vi "Read (Waveform).vi"(5 "Bind Source Channel (2: None)":i32(ring)=2 items=["Sub Source 0", "Sub Source 1", "None"], 7 "Probe atenuation":dbl format="%#_13g", 8 "error in (no error)":errorcluster, 9 "Timeout (10000 ms)":u32=10000, 10 "Source (0: Channel 1)":u16(ring) items=["Channel 1", "Channel 2", "Channel 3", "Channel 4", "Math", "Reference A", "Reference B", "Reference C", "Reference D", "FFT"], 11 "KS EDU-X 1002G in":refnum<class "KS EDU-X 1002G.lvclass">) -> (0 "error out":errorcluster, 2 "Waveform Data":waveform(dbl)(graph), 3 "KS EDU-X 1002G out":refnum<class "KS EDU-X 1002G.lvclass">)   [LabVIEW 2020, in "Oscilloscope.lvlib" / "KS EDU-X 1002G.lvclass"]
uses:
  KS EDU-X 1002G.lvclass
  C:/Users/ronad/Osciloscopio/Osciloscopio DQMH/Libraries/Oscilloscope/Clases/Osciloscopio/Osciloscopio.lvclass
  Clases/Osciloscopio/Osciloscopio.lvclass/Osciloscopio.ctl
  Clases/Osciloscopio/Read COM.vi
  Clases/Osciloscopio/Write COM.vi
  <instrlib>/Agilent 2000 3000 X-Series/Public/Data/Read Waveforms (Single).vi
  <instrlib>/Agilent 2000 3000 X-Series/Agilent 2000 3000 X-Series.lvlib
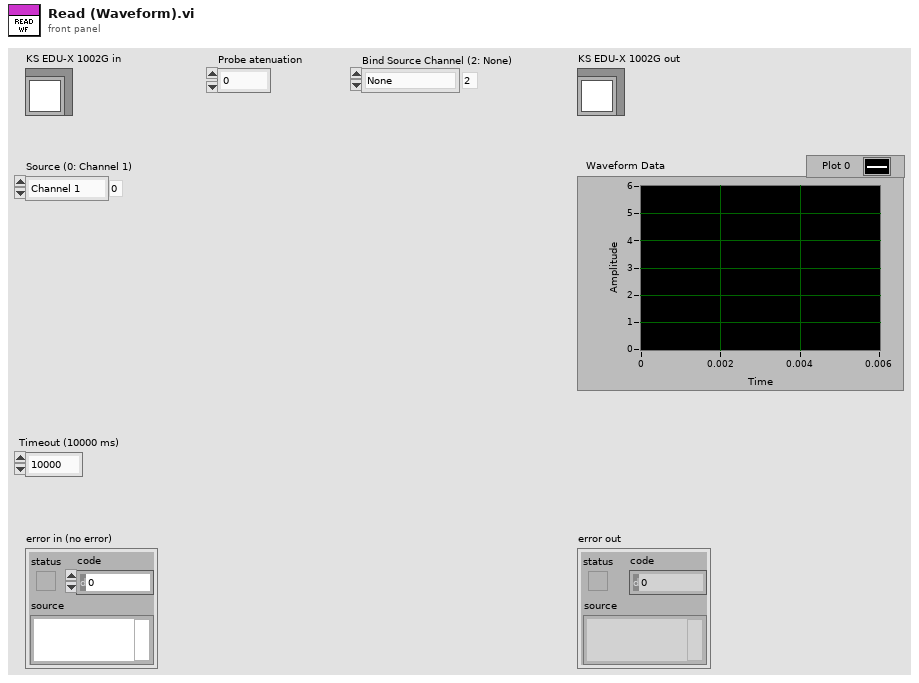
[diagram p1: front panel]
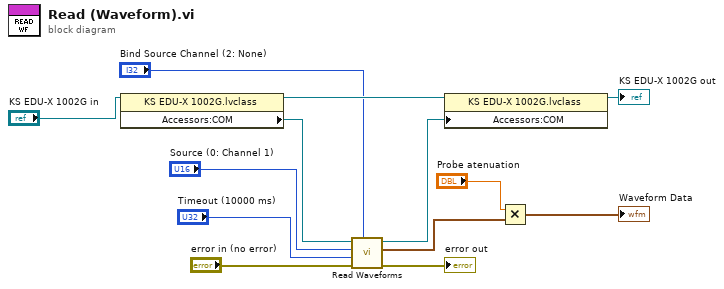
[diagram p0: block diagram]
diagram:
  n1 = property class="KS EDU-X 1002G.lvclass"(reference="KS EDU-X 1002G in") -> (reference out=w10:refnum<class "KS EDU-X 1002G.lvclass">, "Accessors:COM"=w12:refnum<visa-resource-name>)  [unwired: 1 in, 1 out]
  n2 = call-poly <instrlib>:"Read Waveforms.vi"("Bind Source Channel (2: None)"="Bind Source Channel (2: None)", "error in (no error)"="error in (no error)", "Timeout (10000 ms)"="Timeout (10000 ms)", "Source Channel (0: Channel 1)"="Source (0: Channel 1)", "VISA resource name"=w12) -> ("error out"=→"error out":errorcluster, "Waveform Data"=w2:waveform(dbl), "VISA resource name out"=w11:refnum<visa-resource-name>)  [unwired: 4 in]
  n3 = property class="KS EDU-X 1002G.lvclass"(reference=w10, "Accessors:COM"=w11) -> (reference out=→"KS EDU-X 1002G out":refnum<class "KS EDU-X 1002G.lvclass">)  [unwired: 1 in, 1 out]
  n4 = Multiply(x="Probe atenuation", y=w2) -> (x*y=→"Waveform Data":waveform(dbl))
